vi "SendQueryTo8742.vi"(8 "error in (no error)":errorcluster, 10 "Command":string, 11 "PicoMotor8742Comm in":refnum<class "PicoMotor8742Comm.lvclass">) -> (0 "error out":errorcluster, 2 "Reply":string, 3 "PicoMotor8742Comm out":refnum<class "PicoMotor8742Comm.lvclass">)   [LabVIEW 2013, in "PicoMotor8742Comm.lvclass"]
uses:
  PicoMotor8742Comm.lvclass
  PicoMotor8742Comm.lvclass/PicoMotor8742Comm.ctl
  ASCIICommClass.lvclass
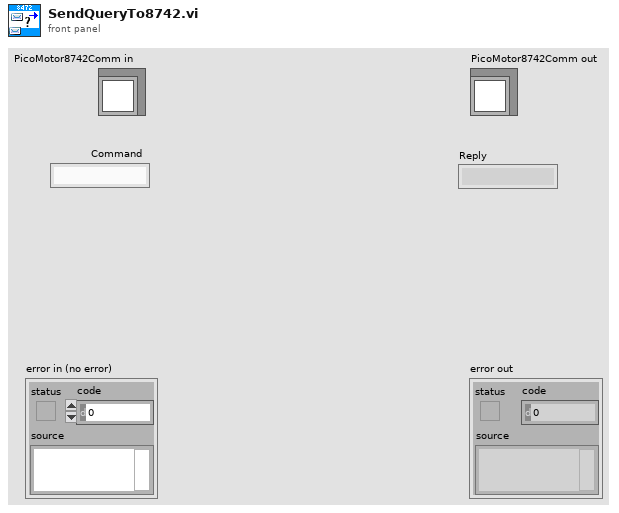
[diagram p1: front panel]
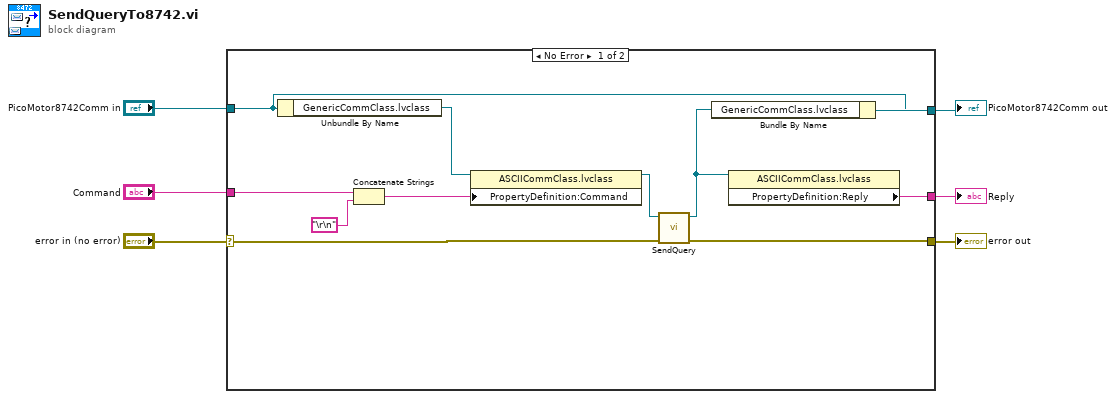
[diagram p0: block diagram]
diagram:
  n1 = case shown="No Error" "error in (no error)" {
    selector: "error in (no error)" -> [w8 w19]
    tunnel: [w7 w19] -> w5
    tunnel: "PicoMotor8742Comm in" -> [w15 w18]
    tunnel: "Command" -> [w16 _]
    tunnel: [w17 w18] -> w2
    tunnel: [w12 _] -> w1
    frame No Error {
      n2 = Unbundle By Name(w15) -> ("GenericCommClass.lvclass"=w14:refnum<class "ASCIICommClass.lvclass">)
      n3 = Concatenate Strings(w16, "\r\n") -> (w13:string)
      n4 = property class="ASCIICommClass.lvclass"(reference=w14, "PropertyDefinition:Command"=w13) -> (reference out=w10:refnum<class "ASCIICommClass.lvclass">)  [unwired: 1 in, 1 out]
      n5 = call-dynamic "SendQuery.vi"("error in (no error)"=w8, "StringCommClass in"=w10) -> ("error out"=w7:errorcluster, "StringCommClass out"=w9:refnum<class "ASCIICommClass.lvclass">)  [unwired: 8 in]
      n6 = Bundle By Name(cluster=w15, "GenericCommClass.lvclass"=w9) -> (w17:refnum<class "PicoMotor8742Comm.lvclass">)
      n7 = property class="ASCIICommClass.lvclass"(reference=w9) -> ("PropertyDefinition:Reply"=w12:string)  [unwired: 1 in, 2 out]
    }
    frame Error {
    }
  }
  "error out" <- w5
  "PicoMotor8742Comm out" <- w2
  "Reply" <- w1
